vi "5.vi"() -> ()   [LabVIEW 2017]
panel:
  out "字符串":string
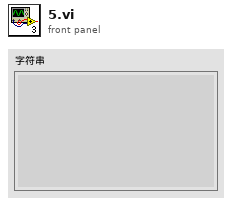
[diagram p1: front panel]
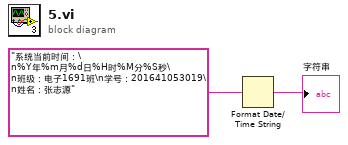
[diagram p0: block diagram]
diagram:
  n1 = Format Date/Time String(time format string (%c)="系统当前时间：\n%Y年%m月%d日%H时%M分%S秒\n班级：电子1691班\n学号：201641053019\n姓名：张志源" ("时间格式字符串(%c)")) -> (date/time string=→"字符串":string)  [unwired: 2 in]
